vi "ConvertWavelengthRange.vi"(2 "error in (no error)":errorcluster, 3 "UserString":string) -> (0 "error out":errorcluster, 1 "Array":dbl[](array[numeric]))   [LabVIEW 2012]
uses:
  <vilib>/regexp/Match Regular Expression.xnode
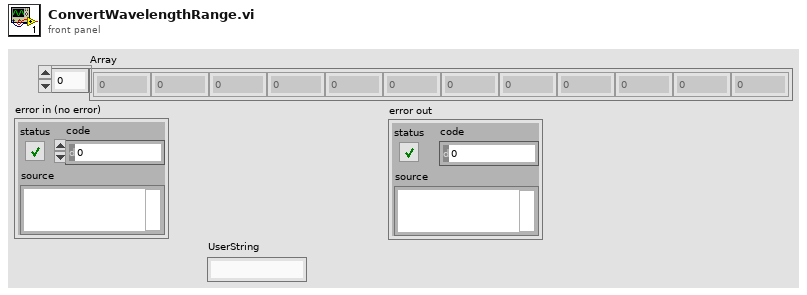
[diagram p1: front panel]
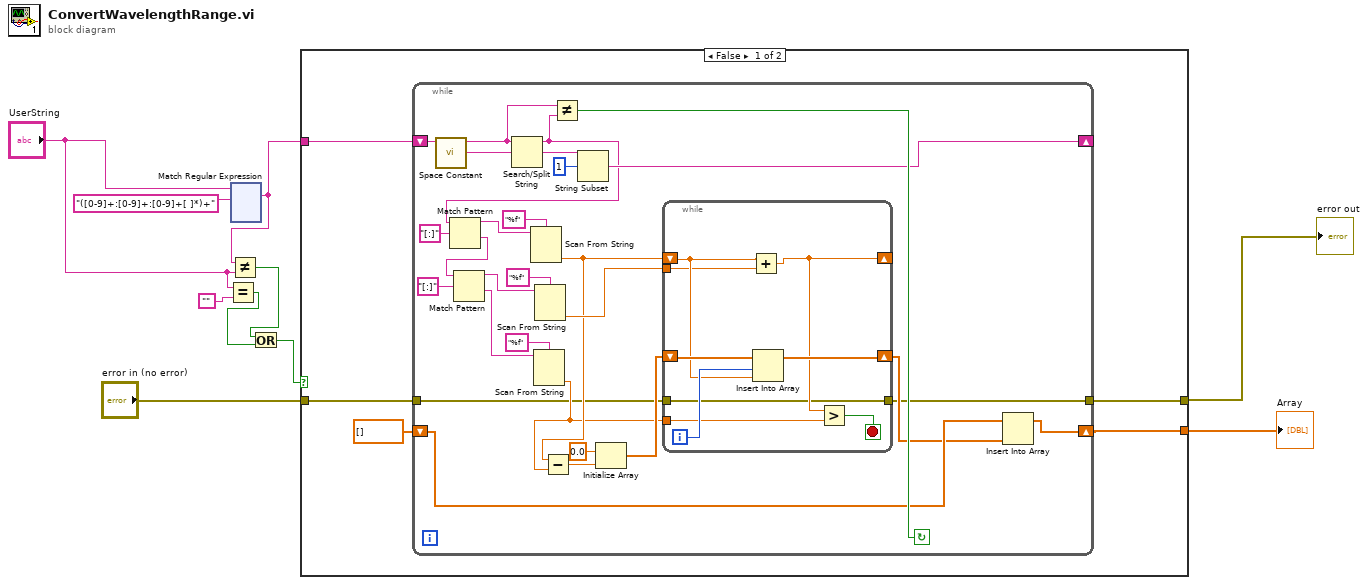
[diagram p0: block diagram]
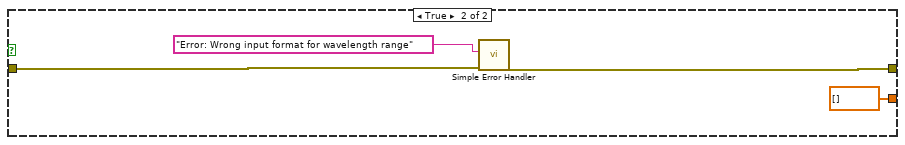
[diagram p2: hidden frame]
diagram:
  n1 = Equal?(x="UserString", y="") -> (x = y?=w1:bool)
  n2 = xnode "Match Regular Expression"("input string"="UserString", "regular expression"="([0-9]+:[0-9]+:[0-9]+[ ]*)+") -> ("whole match"=w7:string)  [unwired: 4 in, 4 out]
  n3 = Not Equal?(x=w7, y="UserString") -> (x != y?=w5:bool)
  n4 = Or(x=w5, y=w1) -> (x .or. y?=w4:bool)
  n5 = case shown="False" w4 {
    tunnel: "error in (no error)" -> [w14 w55]
    tunnel: [w15 w54] -> w8
    tunnel: w7 -> [w13 _]
    tunnel: [w12 dbl[] []] -> w6
    frame False {
      n6 = while {
        shift-right: [w34] -> _
        shift-left: w13 -> [w41]
        shift-right: [w22] -> w12
        shift-left: dbl[] [] -> [w19]
        tunnel: [w17] -> w15
        tunnel: w14 -> [w16]
        stop <- w40 continue-if-true
        n7 = call <vilib>:"Space Constant.vi"() -> ("String"=w42:string)
        n8 = Search/Split String(string=w41, search string/char (-)=w42) -> (substring before match=w23:string, match + rest of string=w38:string)  [unwired: 1 in, 1 out]
        n9 = Match Pattern(string=w23, regular expression="[:]") -> (before substring=w35:string, after substring=w24:string)  [unwired: 1 in, 2 out]
        n10 = Match Pattern(string=w24, regular expression="[:]") -> (before substring=w31:string, after substring=w29:string)  [unwired: 1 in, 2 out]
        n11 = Scan From String(format string="%f", input string=w35) -> (output 1=w21:dbl)  [unwired: 3 in, 3 out]
        n12 = Scan From String(format string="%f", input string=w29) -> (output 1=w20:dbl)  [unwired: 3 in, 3 out]
        n13 = Scan From String(format string="%f", input string=w31) -> (output 1=w25:dbl)  [unwired: 3 in, 3 out]
        n14 = Subtract(x=w21, y=w20) -> (x-y=w28:dbl)
        n15 = Not Equal?(x=w41, y=w23) -> (x != y?=w40:bool)
        n16 = String Subset(string=w38, offset (0)=1) -> (substring=w34:string)  [unwired: 1 in]
        n17 = Initialize Array(0.0 ("element"), w28) -> (w26:dbl[])
        n18 = while {
          shift-right: [w46] -> _
          shift-left: w21 -> [w48]
          shift-right: [w49] -> w18
          shift-left: w26 -> [w51]
          tunnel: w25 -> [w47]
          tunnel: w20 -> [w45]
          tunnel: [w43] -> w17
          tunnel: w16 -> [w43]
          i -> [w50]
          stop <- w44 stop-if-true
          n19 = Add(x=w48, y=w47) -> (x+y=w46:dbl)
          n20 = Insert Into Array(array=w51, index=w50, new element=w48) -> (w49:dbl[])
          n21 = Greater?(x=w46, y=w45) -> (0:w44:bool)
        }
        n22 = Insert Into Array(array=w19, new element=w18) -> (w22:dbl[])  [unwired: 1 in]
      }
    }
    frame True {
      n23 = call <vilib>:"Simple Error Handler.vi"("error source (\" \")"="Error: Wrong input format for wavelength range", "error in (no error)"=w55) -> ("error out"=w54:errorcluster)  [unwired: 3 in, 4 out]
    }
  }
  "Array" <- w6
  "error out" <- w8
